vi "Plot Details Write.vi"(4 "error in (no error)":errorcluster, 5 "Value":T1(array[cluster]), 6 "Container State":T3, 7 "Display State In":T2 {"Time_data" format="%<%.3X>T"}) -> (0 "error out":errorcluster, 3 "Display State Out":T2 {"Time_data" format="%<%.3X>T"})   [LabVIEW 2015, in "2D Buffer Display.xctl"]
doc: "Update the properties of the individual plots:\n* Name - name that will appear on the legend\n* Line Width - 0-5; as in the plot properties dialog\n* Line Style - 0 -4; as defined in the plot properties dialog\n* Line color - use color box constant."
uses:
  2D Buffer Display.xctl
  <vilib>/_xctls/Container State.ctl
  Graph_State.ctl
  <vilib>/_xctls/XControlSupport.lvlib
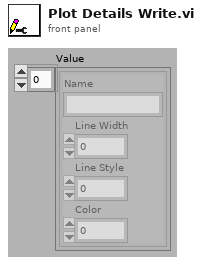
[diagram p1: front panel]
types:
  T1 = cluster{"Name":string, "Line Width":u8, "Line Style":u8, "Color":u32}[]
  T2 = typedef "2D Buffer Display.xctl/Graph_State.ctl" = cluster{"History":u16, "Time_data":timestamp[], "Data_Out":sgl[][][], "Channels":bool[], "Variable":bool[], "Variable Tags":string[], "Channel Tags":string[], "Plot Details":cluster{"Name":string, "Line Width":u8, "Line Style":u8, "Color":u32}[], "Y-Axis Labels":string[], "Avg Data":cluster{"mean":dbl, "standard deviation":dbl}[][]}
  T3 = typedef "XControlSupport.lvlib/Container State.ctl" = cluster{"Indicator?":bool, "Run Mode?":bool, " Refnum":refnum<vi>}
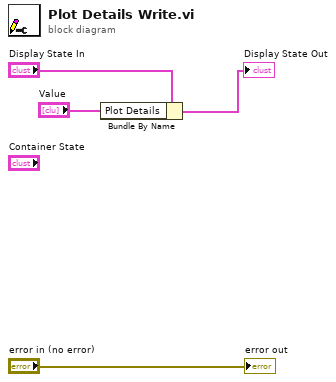
[diagram p0: block diagram]
diagram:
  n1 = Bundle By Name(cluster="Display State In", "Plot Details"="Value") -> (→"Display State Out":T2)
  "error out" <- "error in (no error)"
